vi "Open SQLServer Connection.vi"(5 "Workstation ID":string="VENKY", 7 "Data Source":string="VENKY\\SQLEXPRESS", 8 "error in (no error)":errorcluster, 9 "Password":string, 10 "UserID":string, 11 "DB Name":string) -> (0 "error out":errorcluster, 3 "ADODB._Connection 2":refnum<k7>)   [LabVIEW 2017]
panel:
  in  "ADODB._Connection":refnum<k7>
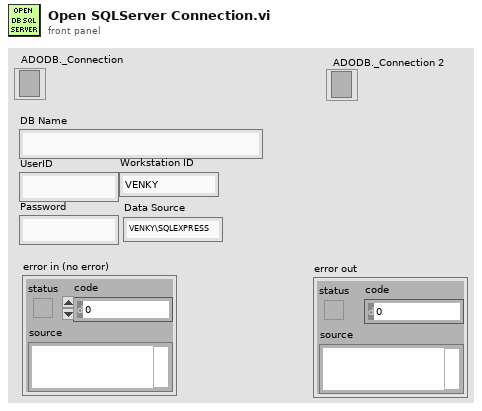
[diagram p1: front panel]
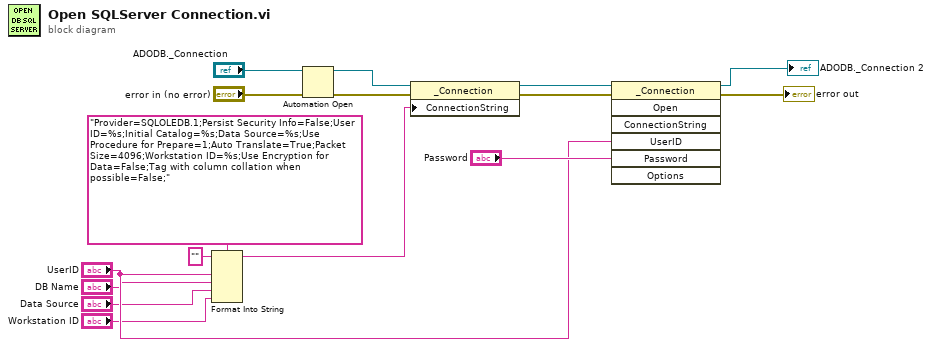
[diagram p0: block diagram]
diagram:
  n1 = Format Into String(format string="Provider=SQLOLEDB.1;Persist Security Info=False;User ID=%s;Initial Catalog=%s;Data Source=%s;Use Procedure for Prepare=1;Auto Translate=True;Packet Size=4096;Workstation ID=%s;Use Encryption for Data=False;Tag with column collation when possible=False;" ("connection information 2"), initial string="", "UserID", "DB Name", "Data Source", "Workstation ID") -> (resulting string=w2:string)  [unwired: 1 in, 1 out]
  n2 = Automation Open(error in (no error)="error in (no error)", Automation Refnum="ADODB._Connection") -> (Automation Refnum=w11:refnum<k7>, error out=w8:errorcluster)  [unwired: 2 out]
  n3 = property class="_Connection"(reference=w11, error in=w8, "ConnectionString"=w2) -> (reference out=w10:refnum<k7>, error out=w9:errorcluster)
  n4 = invoke class="_Connection" method="Open"(reference=w10, error in=w9, "UserID"="UserID", "Password"="Password") -> (reference out=→"ADODB._Connection 2":refnum<k7>, error out=→"error out":errorcluster)  [unwired: 3 in, 5 out]
